vi "AddServo.vi"(8 "error in (no error)":errorcluster, 11 "Data in":T1) -> (0 "error out":errorcluster, 3 "Data out":T1)   [LabVIEW 2023]
uses:
  controls/ServoData.ctl
  <vilib>/Utility/miscctls.llb/LVStringsAndValuesArrayTypeDef_U16.ctl
  controls/UI Data.ctl
panel:
  in  "Cancel Button":bool
  in  "Channel":u16(ring) items=["1"=1, "2"=2, "3"=3, "4"=4, "5"=5]
  in  "Confirm":bool
  in  "Name":string
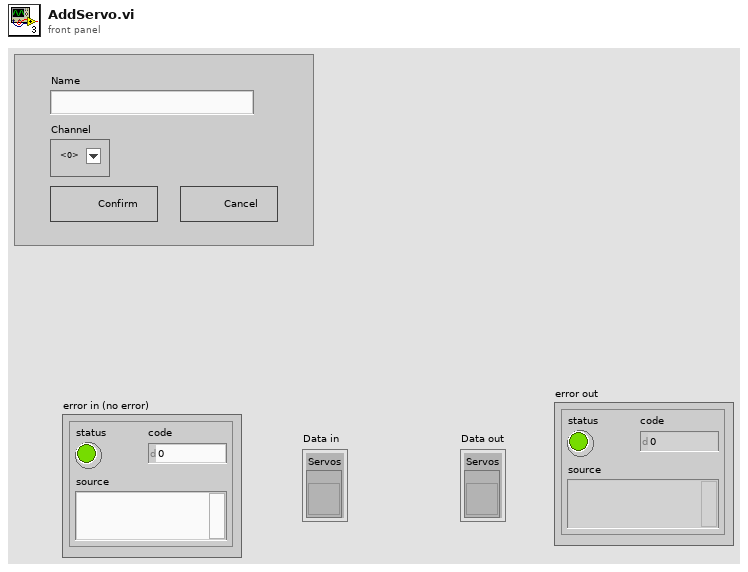
[diagram p1: front panel]
types:
  T1 = typedef "UI Data.ctl" = cluster{"Servos":refnum<vi>}
  T2 = typedef "LVStringsAndValuesArrayTypeDef_U16.ctl" = cluster{"String":string, "Value":u16}[]
  T3 = typedef "ServoData.ctl" = cluster{"Name":string, "Channel":u8, "Delete Button":bool}
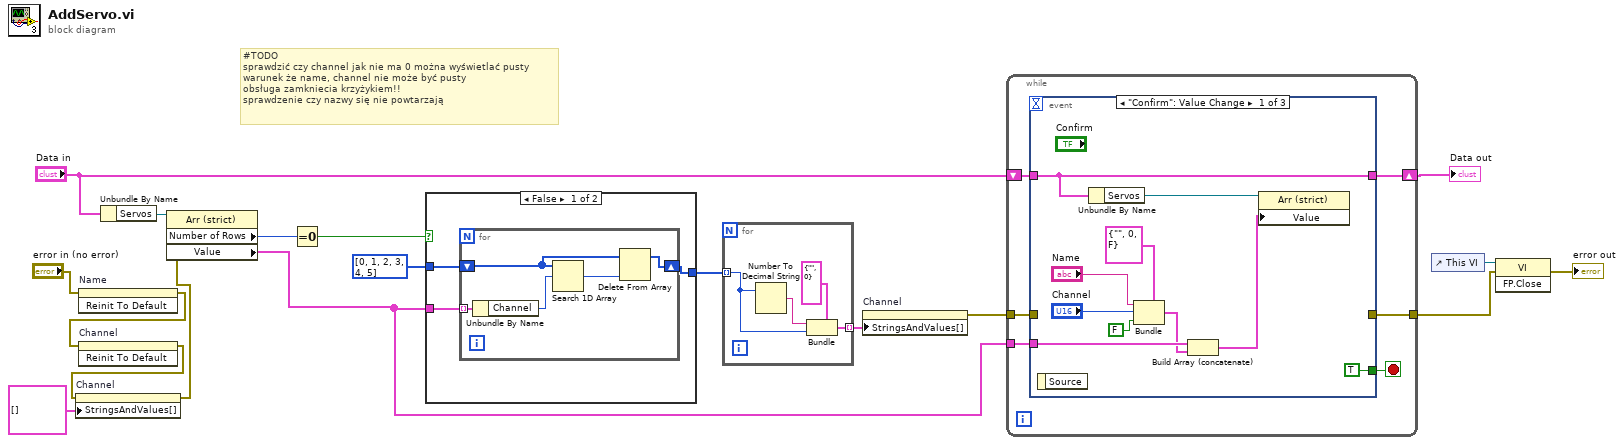
[diagram p0: block diagram]
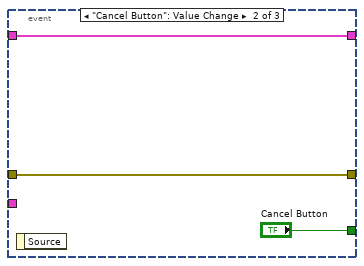
[diagram p2: hidden frame]
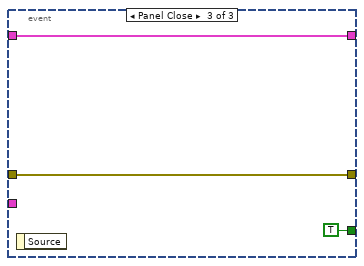
[diagram p3: hidden frame]
diagram:
  # "#TODO\nsprawdzić czy channel jak nie ma 0 można wyświetlać pusty\nwarunek że name, channel nie może być pusty\nobsługa zamkniecia krzyżykiem!!\nsprawdzenie czy nazwy się nie powtarzają"
  n1 = invoke on="Name" class="Str" method="Reinit To Default"(error in="error in (no error)") -> (error out=w5:errorcluster)  [unwired: 2 in, 2 out]
  n2 = invoke on="Channel" class="Ring (strict)" method="Reinit To Default"(error in=w5) -> (error out=w4:errorcluster)  [unwired: 2 in, 2 out]
  n3 = property on="Channel" class="Ring (strict)"(error in=w4, "StringsAndValues[]"=T2 [] ("Strings And Values []")) -> (error out=w3:errorcluster)  [unwired: 1 in, 1 out]
  n4 = Unbundle By Name("Data in") -> ("Servos"=w16:refnum<vi>)
  n5 = property class="Arr (strict)"(reference=w16, error in=w3) -> ("Number of Rows"=w12:u32, "Value"=w1:T3[])  [unwired: 2 out]
  n6 = Equal To 0?(x=w12) -> (x = 0?=w11:bool)
  n7 = case shown="False" w11 {
    tunnel: w1 -> [w21 _]
    tunnel: u8[] [0, 1, 2, 3, 4, 5] -> [w20 w27]
    tunnel: [w19 w27] -> w14
    frame False {
      n8 = for {
        tunnel: w21 -> [w26] mode=indexing
        shift-right: [w22] -> w19
        shift-left: w20 -> [w24]
        n9 = Unbundle By Name(w26) -> ("Channel"=w25:u8)
        n10 = Search 1D Array(1D array=w24, element=w25) -> (index of element=w23:i32)  [unwired: 1 in]
        n11 = Delete From Array(array=w24, index=w23) -> (array with subset deleted=w22:u8[])  [unwired: 1 in, 1 out]
      }
    }
    frame True {
    }
  }
  n12 = for {
    tunnel: w14 -> [w30] mode=indexing
    tunnel: [w28] -> w13 mode=indexing
    n13 = Number To Decimal String(number=w30) -> (decimal integer string=w29:string)  [unwired: 1 in]
    n14 = Bundle(cluster=cluster{string, u16} {"", 0}, w29, w30) -> (w28:cluster{string, u16})
  }
  n15 = property on="Channel" class="Ring (strict)"("StringsAndValues[]"=w13) -> (error out=w8:errorcluster)  [unwired: 2 in, 1 out]
  n16 = while {
    shift-right: [w37] -> w18
    shift-left: "Data in" -> [w36]
    tunnel: w1 -> [w34]
    tunnel: w8 -> [w33]
    tunnel: [w32] -> w7
    stop <- w35 stop-if-true
    n17 = event shown="[0] \"Confirm\": Value Change" {
      selector: _ -> [_ _ _]
      dyn-events: _ -> [_ _ _]
      timeout: _ -> [_ _ _]
      tunnel: [w39 w49 w52] -> w37
      tunnel: w36 -> [w39 w49 w52]
      tunnel: [TRUE ("Cancel Button") "Cancel Button" TRUE ("Cancel Button")] -> w35
      tunnel: w34 -> [w42 _ _]
      tunnel: w33 -> [_ w48 w51]
      tunnel: [_ w48 w51] -> w32
      event "Confirm": Value Change {
        n18 = event-data() -> ()  [unwired: 1 in, 1 out]
        n19 = Unbundle By Name(w39) -> ("Servos"=w40:refnum<vi>)
        n20 = Bundle(cluster=T3 {"Name"="", "Channel"=0, "Delete Button"=FALSE} ("Servo data"), "Name"="Name", "Channel"="Channel", "Delete Button"=FALSE) -> (w41:T3)
        n21 = Build Array (concatenate)(w42, w41) -> (w38:T3[])
        n22 = property class="Arr (strict)"(reference=w40, "Value"=w38) -> ()  [unwired: 1 in, 2 out]
      }
      event "Cancel Button": Value Change {
        n23 = event-data() -> ()  [unwired: 1 in, 1 out]
      }
      event Panel Close {
        n24 = event-data() -> ()  [unwired: 1 in, 1 out]
      }
    }
  }
  "Data out" <- w18
  n25 = control-ref of="This VI"() -> (w10:refnum<vi>)
  n26 = invoke class="VI" method="FP.Close"(reference=w10, error in=w7) -> (error out=→"error out":errorcluster)  [unwired: 1 in, 2 out]
